vi "MH-Obtain Queue.vi"(0 "Initial message":string) -> (4 "MH Queue":refnum<queue>)   [LabVIEW 2020]
uses:
  MH-Message.ctl
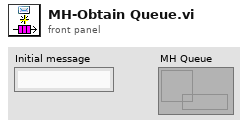
[diagram p1: front panel]
types:
  T1 = typedef "MH-Message.ctl" = cluster{"Message":string, "Data":variant}
  T2 = cluster{"Initial message":string, "Data":variant}
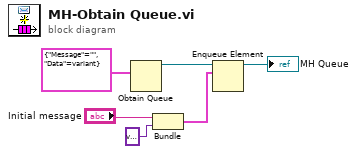
[diagram p0: block diagram]
diagram:
  n1 = Obtain Queue(element data type=T1 {"Message"="", "Data"=variant}) -> (queue out=w4:refnum<queue>)  [unwired: 4 in, 2 out]
  n2 = Bundle("Initial message"="Initial message", "Data"=variant) -> (w5:T2)  [unwired: 1 in]
  n3 = Enqueue Element(queue=w4, element=w5) -> (queue out=→"MH Queue":refnum<queue>)  [unwired: 2 in, 2 out]
